vi "set thread pool.vi"(10 "dispatcher":refnum<data-value>, 11 "task in":refnum<class "task.lvclass">) -> (3 "task out":refnum<class "task.lvclass">)   [LabVIEW 2013, in "task.lvclass"]
uses:
  task.lvclass
  dispatcher/thread pool.lvclass
  task.lvclass/task.ctl
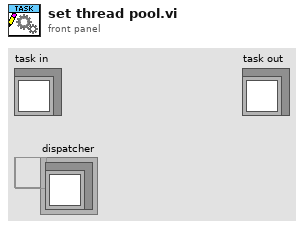
[diagram p1: front panel]
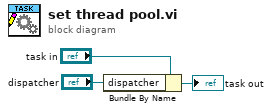
[diagram p0: block diagram]
diagram:
  n1 = Bundle By Name(cluster="task in", "dispatcher"="dispatcher") -> (→"task out":refnum<class "task.lvclass">)
